vi "FT_Read.vi"(8 "error in (no error)":errorcluster, 9 "dwBytestoRead":u32, 11 "ftHandle_in":u32 format="%.0x") -> (0 "error out":errorcluster, 1 "lpBytesReturned":u32, 2 "lpBuffer_out":u8[](array[numeric]) format="%.0x", 3 "ftHandle_out":u32 format="%.0x", 5 "status":u32)   [LabVIEW 2019]
uses:
  FT_Error_codes.vi
  ftd2xx.dll
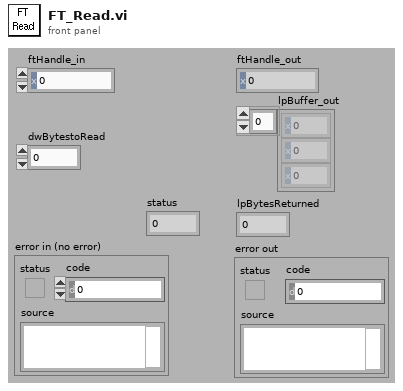
[diagram p1: front panel]
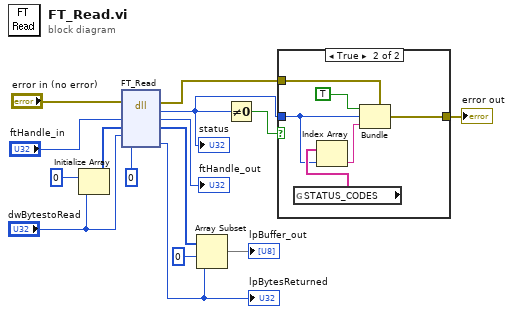
[diagram p0: block diagram]
diagram:
  n1 = Initialize Array(u8 0 ("Numeric"), "dwBytestoRead") -> (w5:u8[])
  n2 = dll-call lib="ftd2xx.dll" fn="FT_Read"(error in="error in (no error)", "ftHandle"="ftHandle_in", "lpBuffer"=w5, "nBufferSize"="dwBytestoRead", "lpBytesWritten"=u32 0 ("lpBytesReturned_in")) -> (error out=w12:errorcluster, "status"=w9:u32, "ftHandle"=→"ftHandle_out":u32, "lpBuffer"=w4:u8[], "lpBytesWritten"=w1:u32)  [unwired: 3 in, 1 out]
  "status" <- w9
  "lpBytesReturned" <- w1
  n3 = Array Subset(array=w4, index=0, length=w1) -> (→"lpBuffer_out":u8[])
  n4 = Not Equal To 0?(x=w9) -> (x != 0?=w10:bool)
  n5 = case shown="True" w10 {
    tunnel: w12 -> [w16 w22]
    tunnel: [w16 w21] -> w11
    tunnel: w9 -> [_ w17]
    frame False {
    }
    frame True {
      n6 = global read "FT_Error_codes.vi" "STATUS_CODES"() -> (w18:string[])
      n7 = Index Array(array=w18, index=w17) -> (element=w19:string)
      n8 = Bundle(cluster=w22, "status"=TRUE, "code"=w17, "source"=w19) -> (w21:errorcluster)
    }
  }
  "error out" <- w11
